vi "Render Layer.vi"(7 "Factor":dbl, 8 "Layer":T1[](array[typedef]), 9 "Textures":string[](array[string]), 10 "Camera":refnum<class "Camera.lvclass">, 11 "Renderer in":refnum<class "Renderer.lvclass">) -> ()   [LabVIEW 2021, in "Galaxy.lvclass"]
uses:
  Galaxy.lvclass
  Camera/Camera.lvclass
  Renderer/Renderer.lvclass
  Re-use Libraries/Vector 2D/Vector 2D.lvclass
  Resource Manager/Resource Manager.lvclass
  Star.ctl
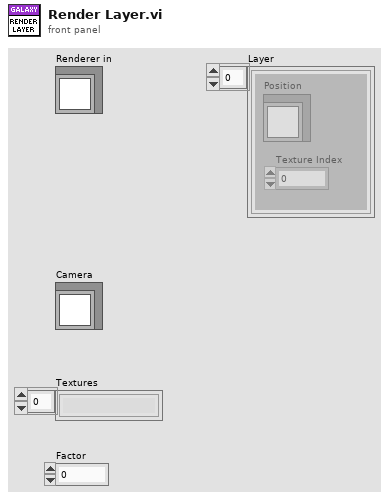
[diagram p1: front panel]
types:
  T1 = typedef "Galaxy.lvclass/Star.ctl" = cluster{"Position":refnum<class "Vector 2D.lvclass">, "Texture Index":i32}
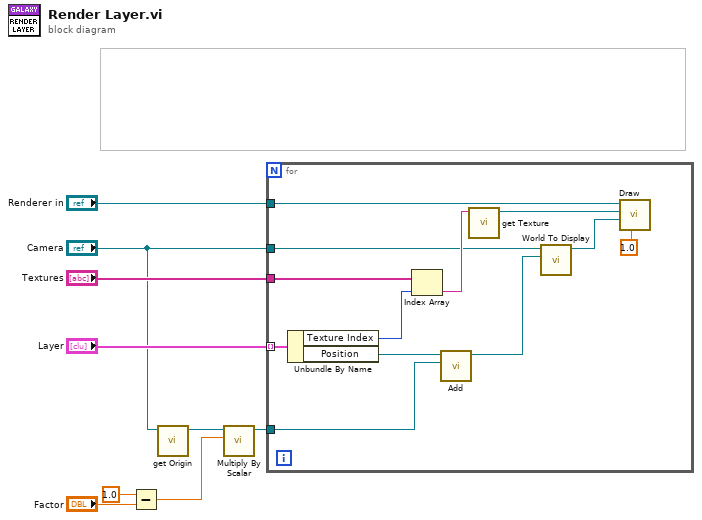
[diagram p0: block diagram]
diagram:
  n1 = Subtract(x=1.0, y="Factor") -> (x-y=w2:dbl)
  n2 = call "get Origin.vi"("Camera in"="Camera") -> ("Origin"=w3:refnum<class "Vector 2D.lvclass">)  [unwired: 10 in]
  n3 = call "Multiply By Scalar.vi"("x"=w2, "A"=w3) -> ("Ax"=w1:refnum<class "Vector 2D.lvclass">)  [unwired: 9 in]
  n4 = for {
    tunnel: "Layer" -> [w20] mode=indexing
    tunnel: "Renderer in" -> [w19]
    tunnel: "Textures" -> [w18]
    tunnel: "Camera" -> [w16]
    tunnel: w1 -> [w12]
    n5 = Unbundle By Name(w20) -> ("Texture Index"=w15:i32, "Position"=w11:refnum<class "Vector 2D.lvclass">)
    n6 = Index Array(array=w18, index=w15) -> (element=w17:string)
    n7 = call "Add.vi"("B"=w12, "A"=w11) -> ("A+B"=w10:refnum<class "Vector 2D.lvclass">)  [unwired: 9 in]
    n8 = call "get Texture.vi"("Texture Name"=w17) -> ("Texture"=w21:refnum<class "Texture.lvclass">)  [unwired: 10 in]
    n9 = call "World To Display.vi"("World Position"=w10, "Camera in"=w16) -> ("Display Position"=w13:refnum<class "Vector 2D.lvclass">)  [unwired: 9 in]
    n10 = call "Draw.vi"("Scale"=sgl 1.0, "Destination"=w13, "Texture"=w21, "Renderer"=w19) -> ()  [unwired: 7 in, 1 out]
  }
